vi "watermark subset.vi"() -> ()   [LabVIEW 2009]
uses:
  <vilib>/picture/picture.llb/Draw True-Color Pixmap.vi
panel:
  in  "rectangle corner":cluster{"x":i16, "y":i16}
  in  "watermark":bool[][](array[boolean])
  in  "picture":picture
  in  "invert?":bool
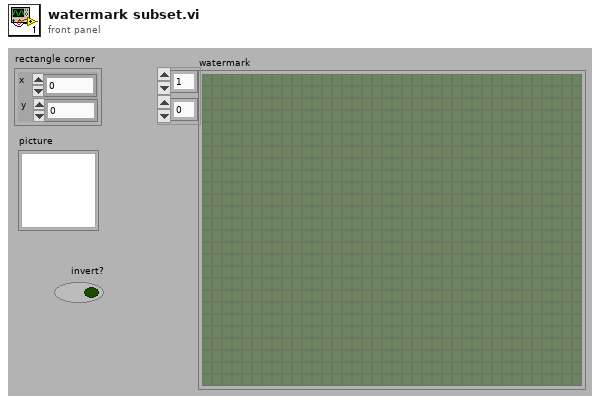
[diagram p1: front panel]
types:
  T1 = cluster{"left":i16, "top":i16, "right":i16, "bottom":i16}
  T2 = typedef "imagedata.ctl" = cluster{"image type":i32, "image depth":i32, "image":u8[], "mask":u8[], "colors":u32[], "Rectangle":cluster{"left":i16, "top":i16, "right":i16, "bottom":i16}}
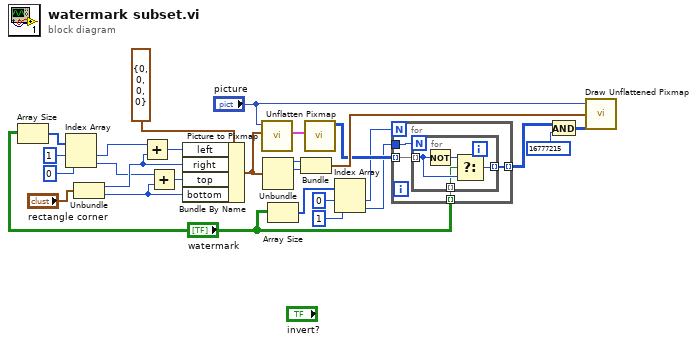
[diagram p0: block diagram]
diagram:
  n1 = Array Size(array="watermark") -> (size(s)=w25:i32[])
  n2 = Index Array(array=w25, index #1=1 ("index"), index #2=0 ("index")) -> (element #1=w18:i32, element #2=w19:i32)
  n3 = Unbundle("rectangle corner") -> ("x"=w20:i16, "y"=w21:i16)
  n4 = Add(x=w18, y=w20) -> (x+y=w17:i32)
  n5 = Add(x=w19, y=w21) -> (x+y=w16:i32)
  n6 = Bundle By Name(cluster=T1 {"left"=0, "top"=0, "right"=0, "bottom"=0} ("subset rect"), "left"=w17, "right"=w20, "top"=w16, "bottom"=w21) -> (w11:T1)
  n7 = call <vilib>:"Picture to Pixmap.vi"("rect"=w11, "picture"="picture") -> ("image data"=w13:T2)  [unwired: 8 in, 1 out]
  n8 = Unbundle(w11) -> ("left"=w12:i16, "top"=w10:i16)  [unwired: 2 out]
  n9 = Array Size(array="watermark") -> (size(s)=w6:i32[])
  n10 = Bundle("left"=w12, "top"=w10) -> (w9:cluster{"left":i16, "top":i16})  [unwired: 1 in]
  n11 = call <vilib>:"Unflatten Pixmap.vi"("image data"=w13) -> ("24-bit pixmap"=w8:u32[][])  [unwired: 4 in, 6 out]
  n12 = Index Array(array=w6, index #1=0 ("index"), index #2=1 ("index")) -> (element #1=w2:i32, element #2=w1:i32)
  n13 = for {
    N: w2 -> [_]
    tunnel: w8 -> [w31] mode=indexing
    tunnel: [w30] -> w7 mode=indexing
    tunnel: "watermark" -> [w29] mode=indexing
    tunnel: w1 -> [w28]
    n14 = for {
      N: w28 -> [_]
      tunnel: w31 -> [w34] mode=indexing
      tunnel: [w33] -> w30 mode=indexing
      tunnel: w29 -> [w32] mode=indexing
      n15 = Not(x=w34) -> (.not. x?=w35:u32)
      n16 = Select(t=w35, s=w32, f=w34) -> (s? t:f=w33:u32)
    }
  }
  n17 = And(x=w7, y=u32 16777215) -> (x .and. y?=w14:u32[][])
  n18 = call-poly <vilib>:"Draw Unflattened Pixmap.vi"("picture"="picture", "top left point(0, 0)"=w9, "data (RGB format)"=w14) -> ()  [unwired: 6 in, 1 out]
